vi "Append.vi"(8 "error in (no error)":errorcluster, 9 "Runnable":refnum<class "Runnable.lvclass">, 10 "Name":string, 11 "LUnit Test Suite V2 in":refnum<class "LUnit Test Suite V2.lvclass">) -> (0 "error out":errorcluster, 3 "LUnit Test Suite V2 out":refnum<class "LUnit Test Suite V2.lvclass">)   [LabVIEW 2020, in "LUnit Test Suite V2.lvclass"]
uses:
  LUnit Test Suite V2.lvclass
  Run/Runnable.lvclass
  LUnit Test Suite V2.lvclass/LUnit Test Suite V2.ctl
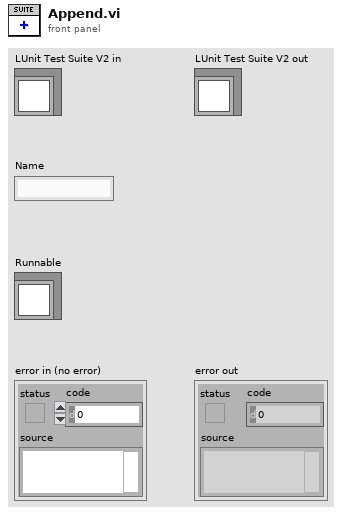
[diagram p1: front panel]
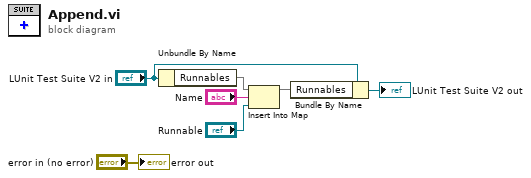
[diagram p0: block diagram]
diagram:
  n1 = Unbundle By Name("LUnit Test Suite V2 in") -> ("Runnables"=w4:map{string, refnum<class "Runnable.lvclass">})
  n2 = Insert Into Map(map in=w4, key="Name", value="Runnable") -> (map out=w3:map{string, refnum<class "Runnable.lvclass">})  [unwired: 2 out]
  n3 = Bundle By Name(cluster="LUnit Test Suite V2 in", "Runnables"=w3) -> (→"LUnit Test Suite V2 out":refnum<class "LUnit Test Suite V2.lvclass">)
  "error out" <- "error in (no error)"
